vi "Chebyeval.vi"(8 "end":dbl=1.0, 9 "start":dbl, 10 "C":dbl[](array[numeric]), 11 "number of points":u32=5) -> (2 "X":dbl[](array[numeric]), 3 "Y":dbl[](array[numeric]))   [LabVIEW 2019]
uses:
  <vilib>/gmath/NI_Gmath.lvlib
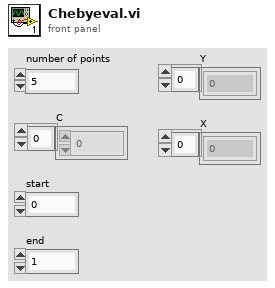
[diagram p1: front panel]
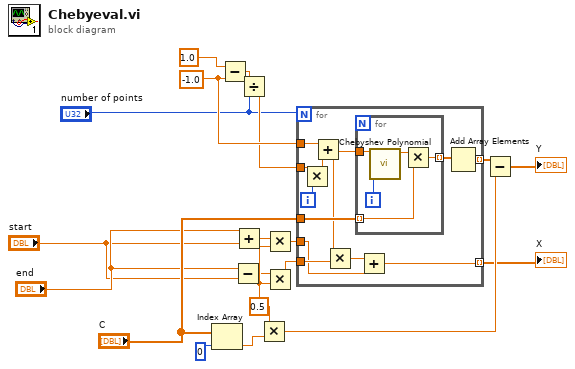
[diagram p0: block diagram]
diagram:
  w10 = 0.5
  w13 = -1.0
  n1 = Index Array(array="C", index=0) -> (element=w15:dbl)
  n2 = Subtract(x=1.0, y=w13) -> (x-y=w17:dbl)
  n3 = Subtract(x="end", y="start") -> (x-y=w9:dbl)
  n4 = Add(x="end", y="start") -> (x+y=w11:dbl)
  n5 = Divide(x=w17, y="number of points") -> (x/y=w12:dbl)
  n6 = Multiply(x=w10, y=w15) -> (x*y=w19:dbl)
  n7 = Multiply(x=w11, y=w10) -> (x*y=w8:dbl)
  n8 = Multiply(x=w9, y=w10) -> (x*y=w7:dbl)
  n9 = for {
    N: "number of points" -> [_]
    tunnel: w12 -> [w31]
    tunnel: w13 -> [w29]
    tunnel: "C" -> [w27]
    tunnel: [w25] -> w18 mode=indexing
    tunnel: [w20] -> w1 mode=indexing
    tunnel: w8 -> [w21]
    tunnel: w7 -> [w23]
    i -> [w30]
    n10 = Multiply(x=w31, y=w30) -> (x*y=w28:dbl)
    n11 = Add(x=w29, y=w28) -> (x+y=w24:dbl)
    n12 = Multiply(x=w24, y=w23) -> (x*y=w22:dbl)
    n13 = for {
      tunnel: w24 -> [w33]
      tunnel: w27 -> [w35] mode=indexing
      tunnel: [w34] -> w26 mode=indexing
      i -> [w32]
      n14 = call <vilib>:"Chebyshev Polynomial.vi"("n"=w32, "x"=w33) -> ("T(n,x)"=w36:dbl)
      n15 = Multiply(x=w36, y=w35) -> (x*y=w34:dbl)
    }
    n16 = Add(x=w22, y=w21) -> (x+y=w20:dbl)
    n17 = Add Array Elements(numeric array=w26) -> (sum=w25:dbl)
  }
  "X" <- w1
  n18 = Subtract(x=w18, y=w19) -> (x-y=→"Y":dbl[])
